vi "IPC-ModbusSerial-ReadCoils.vi"(4 "parity (Even)":u16(ring)=2 caption="奇偶（偶）" items=["无", "奇", "偶"], 5 "baud rate (9600)":u32=9600 caption="波特率(9600)", 6 "VISA resource name":refnum<visa-resource-name>="COM3" caption="VISA资源名称", 7 "error in (no error)":errorcluster caption="错误输入（无错误）", 8 "number of coils":u16 caption="线圈数量", 9 "starting address":u16 caption="起始地址", 10 "unit ID":u8=1 caption="单元ID") -> (0 "error out":errorcluster caption="错误输出", 3 "coil values":bool[](array[boolean]) caption="线圈值")   [LabVIEW 2014]
uses:
  <vilib>/Modbus/master/Create Master Instance (Serial).vi
  <vilib>/Modbus/master/Modbus Master.lvclass
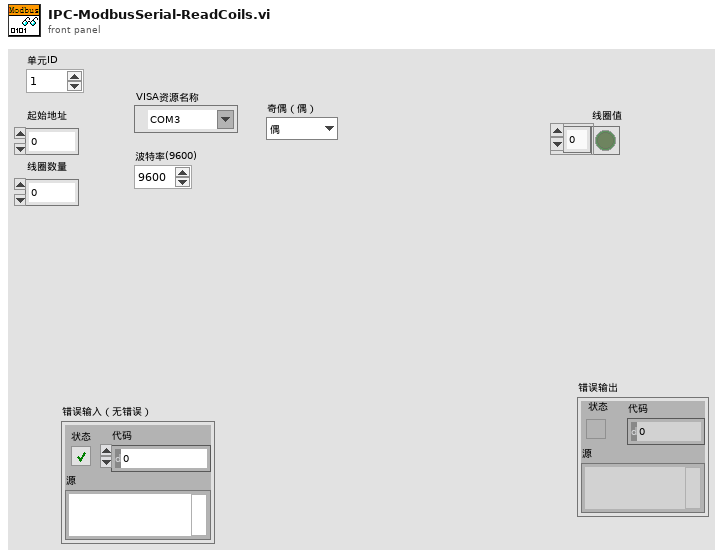
[diagram p1: front panel]
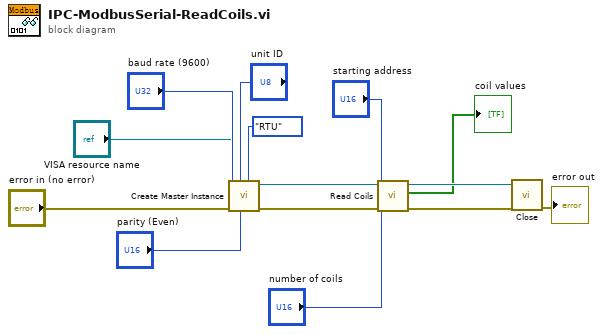
[diagram p0: block diagram]
diagram:
  n1 = call-poly <vilib>:"Create Master Instance.vi"("serial type"=enum16{"RTU", "ASCII"}."RTU", "parity (Even)"="parity (Even)", "unit ID"="unit ID", "error in (no error)"="error in (no error)", "baud rate (9600)"="baud rate (9600)", "VISA resource name"="VISA resource name") -> ("error out"=w6:errorcluster, "serial master instance"=w7:refnum<class "Modbus Master.lvclass">)  [unwired: 4 in]
  n2 = call-dynamic "Read Coils.vi"("error in (no error)"=w6, "number of coils"="number of coils", "starting address"="starting address", "Modbus master in"=w7) -> ("error out"=w4:errorcluster, "coil values"=→"coil values":bool[], "Modbus master out"=w5:refnum<class "Modbus Master.lvclass">)  [unwired: 5 in]
  n3 = call-dynamic "Close.vi"("error in (no error)"=w4, "Modbus master in"=w5) -> ("error out"=→"error out":errorcluster)  [unwired: 9 in]
